vi "Name Tab Control.vi"(9 "TabCtl Refnum":refnum<vi>, 11 "String":string) -> ()   [LabVIEW 2013]
doc: "Jean-Marc Simard \nExaprom inc. 2009"
panel:
  out "error out":errorcluster
  out "Numeric":i32
  out "String[ ]":string[](array[string])
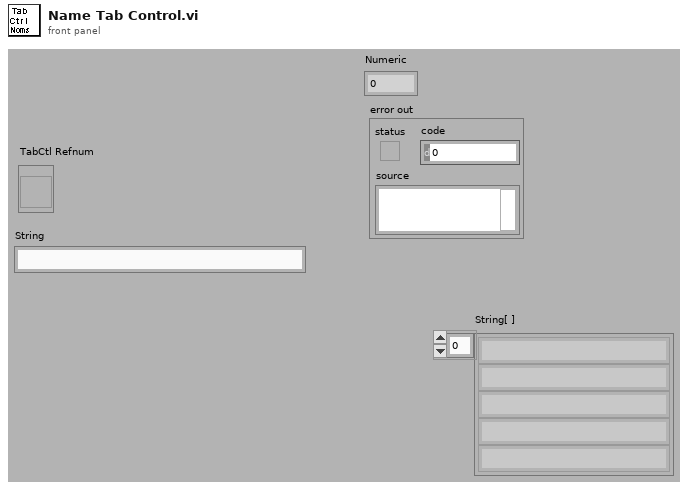
[diagram p1: front panel]
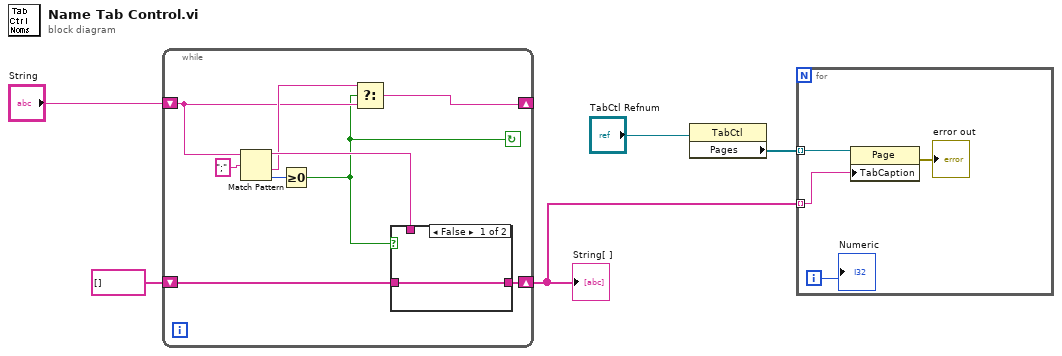
[diagram p0: block diagram]
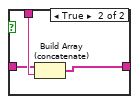
[diagram p2: hidden frame]
diagram:
  n1 = while {
    shift-right: [w12] -> _
    shift-left: "String" -> [w7]
    shift-right: [w9] -> w1
    shift-left: string[] [] ("String[ ]") -> [w10]
    stop <- w6 continue-if-true
    n2 = Match Pattern(string=w7, regular expression=";") -> (before substring=w11:string, after substring=w8:string, offset past match=w13:i32)  [unwired: 2 out]
    n3 = Greater Or Equal To 0?(x=w13) -> (x >= 0?=w6:bool)
    n4 = Select(t=w8, s=w6, f=w7) -> (s? t:f=w12:string)
    n5 = case shown="False" w6 {
      tunnel: w11 -> [_ w18]
      tunnel: w10 -> [w15 w17]
      tunnel: [w15 w16] -> w9
      frame False {
      }
      frame True {
        n6 = Build Array (concatenate)(w17, w18) -> (w16:string[])
      }
    }
  }
  "String[ ]" <- w1
  n7 = property class="TabCtl"(reference="TabCtl Refnum") -> ("Pages"=w2:refnum<vi>[])  [unwired: 1 in, 2 out]
  n8 = for {
    tunnel: w2 -> [w22] mode=indexing
    tunnel: w1 -> [w21] mode=indexing
    i -> [w20]
    n9 = property class="Page"(reference=w22, "TabCaption"=w21) -> (error out=→"error out":errorcluster)  [unwired: 1 in, 1 out]
    "Numeric" <- w20
  }
